vi "uTTA_ReadFileFromMemory_Save.vi"(6 "Last Line":refnum<vi>, 8 "error in":errorcluster, 9 "File Path":path, 10 "Filename":string, 11 "VISA Refnum in":refnum<visa-resource-name>) -> (0 "error out":errorcluster, 1 "Timeout Expanded":bool, 2 "Received":string, 3 "VISA Refnum out":refnum<visa-resource-name>, 4 "Read took ms":i32)   [LabVIEW 2021]
panel:
  out "lowercase file extension":string
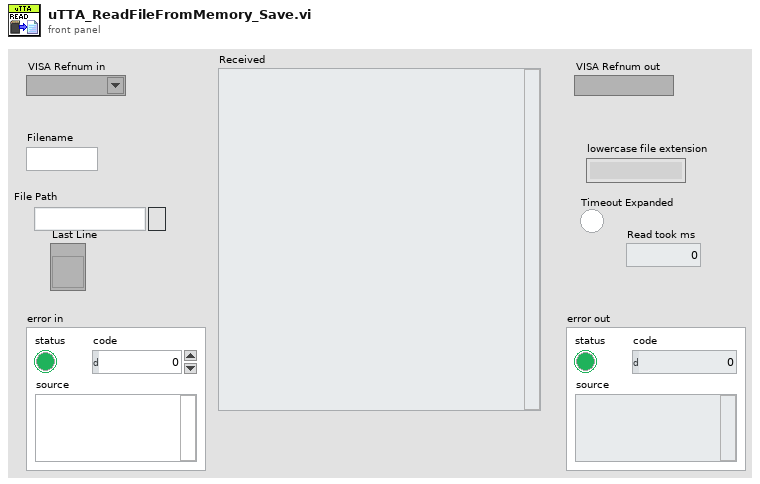
[diagram p1: front panel]
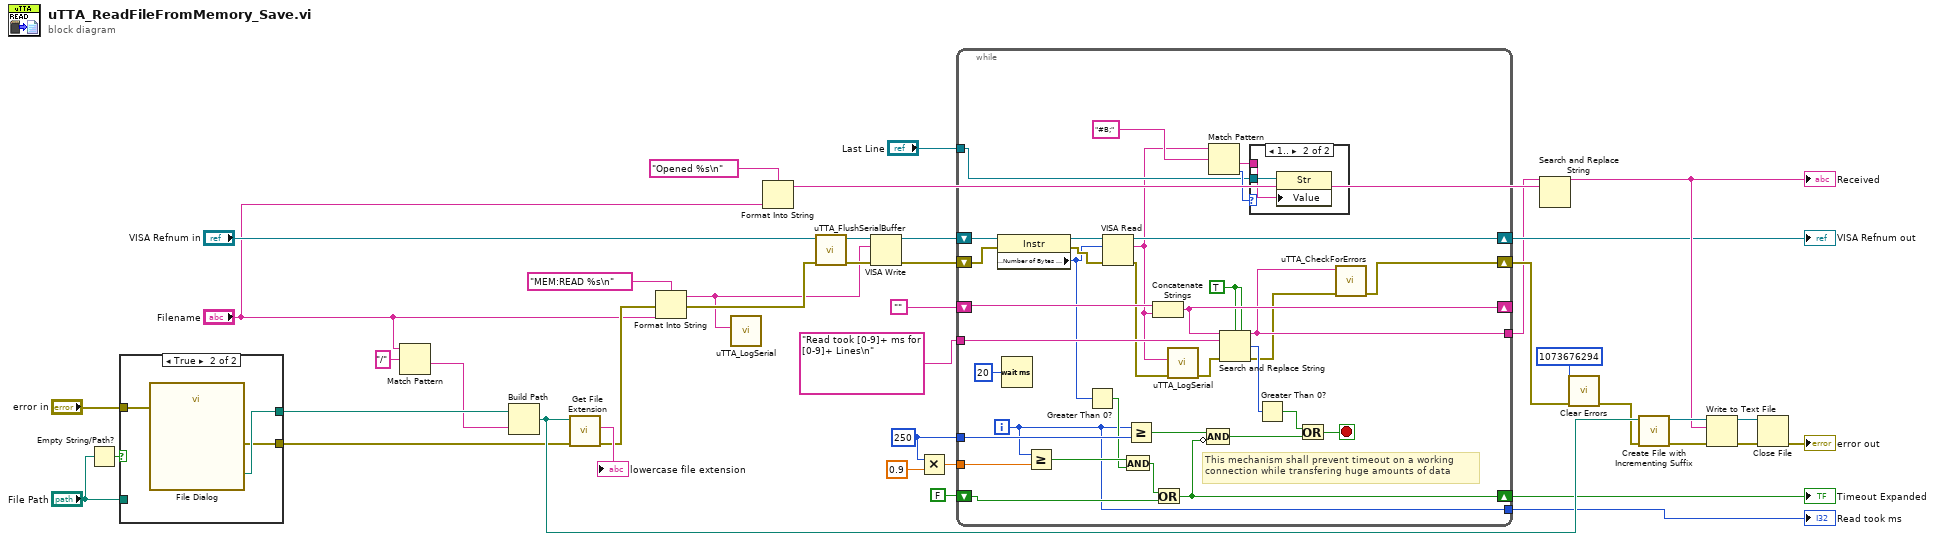
[diagram p0: block diagram]
diagram:
  w11 = 250 ("Timeout(ms)")
  n1 = Empty String/Path?(string/path="File Path") -> (empty?=w40:bool)
  n2 = case shown="True" w40 {
    tunnel: "File Path" -> [w43 _]
    tunnel: [w43 w46] -> w32
    tunnel: "error in" -> [w42 w45]
    tunnel: [w42 w44] -> w29
    frame False {
    }
    frame True {
      n3 = call "File Dialog"("error in"=w45) -> ("selected path"=w46:path, "error out"=w44:errorcluster)  [unwired: 11 in, 2 out]
    }
  }
  n4 = Match Pattern(string="Filename", regular expression="/") -> (after substring=w3:string)  [unwired: 1 in, 3 out]
  n5 = Build Path(base path=w32, name or relative path=w3) -> (appended path=w31:path)
  n6 = call <vilib>:"Get File Extension.vi"("error in (no error)"=w29, "file"=w31) -> ("error out"=w28:errorcluster, "lowercase file extension"=→"lowercase file extension":string)  [unwired: 5 in, 3 out]
  n7 = Format Into String(format string="MEM:READ %s\n", error in=w28, "Filename") -> (resulting string=w1:string, error out=w16:errorcluster)  [unwired: 1 in]
  n8 = call "uTTA_LogSerial.vi"("Data_Sent"=w1) -> ()  [unwired: 6 in, 1 out]
  n9 = Format Into String(format string="Opened %s\n" ("RX Termination(\\n)"), "Filename") -> (resulting string=w26:string)  [unwired: 2 in, 1 out]
  n10 = call "uTTA_FlushSerialBuffer.vi"("error in (no error)"=w16, "VISA Refnum in"="VISA Refnum in") -> ("error out"=w24:errorcluster, "VISA Refnum out"=w23:refnum<visa-resource-name>)  [unwired: 4 in]
  n11 = VISA Write(VISA resource name=w23, write buffer=w1, error in (no error)=w24) -> (VISA resource name out=w20:refnum<visa-resource-name>, error out=w21:errorcluster)  [unwired: 1 out]
  n12 = Multiply(x=w11, y=0.9) -> (x*y=w9:dbl)
  n13 = while {
    shift-right: [w75] -> _
    shift-left: "" -> [w76]
    tunnel: [w67] -> w12
    shift-right: [w65] -> w18
    shift-left: w21 -> [w79]
    shift-right: [w72] -> w14
    shift-left: w20 -> [w80]
    tunnel: w11 -> [w69]
    tunnel: "Read took [0-9]+ ms for [0-9]+ Lines\n" ("RX Termination(\\n)") -> [w68]
    tunnel: w9 -> [w63]
    shift-right: [w57] -> w7
    shift-left: FALSE ("ignore case? (F)") -> [w58]
    tunnel: [w54] -> w6
    tunnel: "Last Line" -> [w51]
    i -> [w54]
    stop <- w70 stop-if-true
    w64 = TRUE ("ignore case? (F)")
    # "This mechanism shall prevent timeout on a working\nconnection while transfering huge amounts of data"
    n14 = property class="Instr"(reference=w80, error in=w79) -> (reference out=w78:refnum<visa-resource-name>, error out=w77:errorcluster, "Serial Settings:Number of Bytes at Serial Port"=w61:u32)
    n15 = Wait (ms)(milliseconds to wait=u32 20) -> ()  [unwired: 1 out]
    n16 = Greater Or Equal?(x=w54, y=w63) -> (x >= y?=w62:bool)
    n17 = Greater Than 0?(x=w61) -> (x > 0?=w60:bool)
    n18 = VISA Read(VISA resource name=w78, byte count=w61, error in (no error)=w77) -> (VISA resource name out=w72:refnum<visa-resource-name>, read buffer=w49:string, error out=w48:errorcluster)  [unwired: 1 out]
    n19 = And(x=w62, y=w60) -> (x .and. y?=w59:bool)
    n20 = Greater Or Equal?(x=w54, y=w69) -> (x >= y?=w56:bool)
    n21 = Concatenate Strings(w76, w49) -> (w75:string)
    n22 = Or(x=w59, y=w58) -> (x .or. y?=w57:bool)
    n23 = call "uTTA_LogSerial.vi"("error in"=w48, "Data_Sent"=w49) -> ("error out"=w47:errorcluster)  [unwired: 5 in]
    n24 = Compound Arithmetic op=AND(w56, invert w57) -> (w55:bool)
    n25 = Match Pattern(string=w49, regular expression="#B;" ("search string")) -> (after substring=w53:string, offset past match=w52:i32)  [unwired: 1 in, 2 out]
    n26 = Search and Replace String(case sensitive?=w64, multiline?=w64, input string=w75, search string=w68, error in=w47) -> (result string=w67:string, number of replacements=w74:i32, error out=w66:errorcluster)  [unwired: 3 in, 1 out]
    n27 = case shown="1.." w52 {
      tunnel: w51 -> [_ w82]
      tunnel: w53 -> [_ w81]
      frame 0, Default {
      }
      frame 1.. {
        n28 = property class="Str"(reference=w82, "Value"=w81) -> ()  [unwired: 1 in, 2 out]
      }
    }
    n29 = Greater Than 0?(x=w74) -> (x > 0?=w71:bool)
    n30 = Or(x=w71, y=w55) -> (x .or. y?=w70:bool)
    n31 = call "uTTA_CheckForErrors.vi"("error in"=w66, "Received"=w67) -> ("error out"=w65:errorcluster)  [unwired: 9 in]
  }
  "VISA Refnum out" <- w14
  "Timeout Expanded" <- w7
  "Read took ms" <- w6
  n32 = Search and Replace String(input string=w12, search string=w26) -> (result string=w25:string)  [unwired: 6 in, 3 out]
  "Received" <- w25
  n33 = call <vilib>:"Clear Errors.vi"("error in (no error)"=w18, "specific error code to clear (0: all)"=1073676294) -> ("error out"=w13:errorcluster)  [unwired: 4 in, 1 out]
  n34 = call <vilib>:"Create File with Incrementing Suffix.vi"("error in (no error)"=w13, "file path"=w31) -> ("error out"=w37:errorcluster, "refnum out"=w36:refnum<file>)  [unwired: 7 in, 1 out]
  n35 = Write to Text File(file (use dialog)=w36, text=w25, error in=w37) -> (refnum out=w34:refnum<file>, error out=w35:errorcluster)  [unwired: 1 in, 1 out]
  n36 = Close File(refnum=w34, error in=w35) -> (error out=→"error out":errorcluster)  [unwired: 1 out]
